vi "Verify Type.vi"(8 "error in (no error)":errorcluster, 11 "CIF_CIPC_Universal in":refnum<class "CIF_CIPC_Universal.lvclass">) -> (0 "error out":errorcluster, 3 "CIF_CIPC_Universal out":refnum<class "CIF_CIPC_Universal.lvclass">)   [LabVIEW 2021, in "CIF_CIPC_Universal.lvclass"]
uses:
  CIF_CIPC_Universal.lvclass
  CIF_CIPC_Universal.lvclass/CIF_CIPC_Universal.ctl
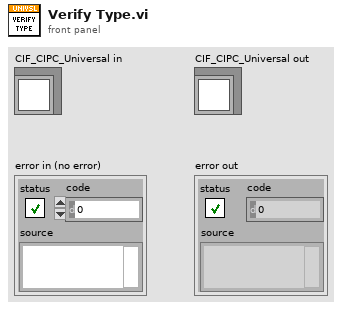
[diagram p1: front panel]
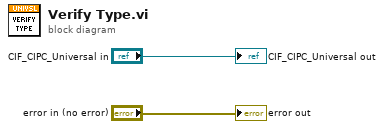
[diagram p0: block diagram]
diagram:
  "error out" <- "error in (no error)"
  "CIF_CIPC_Universal out" <- "CIF_CIPC_Universal in"
